vi "_085.vi"() -> ()   [LabVIEW 2024]
panel:
  out "s? t:f 2":i32
  out "s? t:f":i32
  # "Fundamentals :"
  # "14~>After running this VI,what is the value displayed in the o/p ?"
  # "Nrml Approach :"
  # "Dfrnt Approach :"
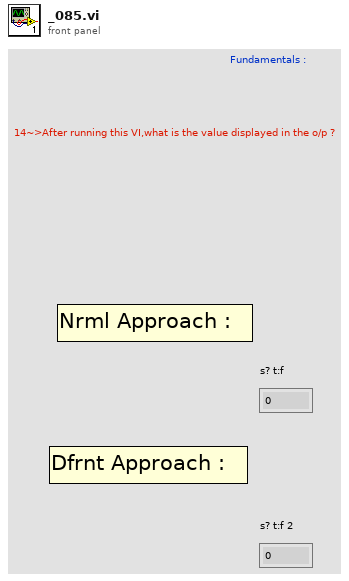
[diagram p1: front panel]
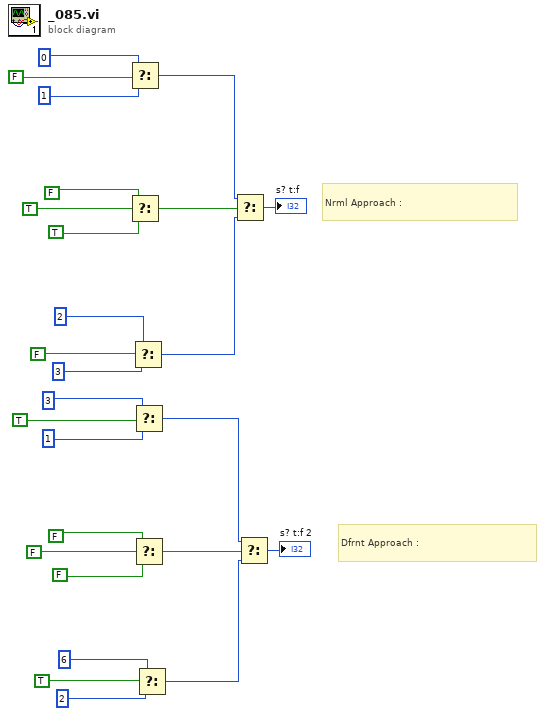
[diagram p0: block diagram]
diagram:
  # "Dfrnt Approach :"
  # "Nrml Approach :"
  n1 = Select(t=0, s=FALSE, f=1) -> (s? t:f=w17:i32)
  n2 = Select(t=FALSE, s=TRUE, f=TRUE) -> (s? t:f=w16:bool)
  n3 = Select(t=2, s=FALSE, f=3) -> (s? t:f=w18:i32)
  n4 = Select(t=3, s=TRUE, f=1) -> (s? t:f=w10:i32)
  n5 = Select(t=FALSE, s=FALSE, f=FALSE) -> (s? t:f=w11:bool)
  n6 = Select(t=6, s=TRUE, f=2) -> (s? t:f=w9:i32)
  n7 = Select(t=w17, s=w16, f=w18) -> (s? t:f=→"s? t:f":i32)
  n8 = Select(t=w10, s=w11, f=w9) -> (s? t:f=→"s? t:f 2":i32)
